vi "ep_Read Current Channels.vi"(8 "error in (no error)":errorcluster, 11 "system info in":refnum<class "EP System Info.lvclass">) -> (0 "error out":errorcluster, 2 "current channels":T1[](array[typedef]) {"physical channels"."channel phase" items=["Phase A (L1)", "Phase B (L2)", "Phase C (L3)", "Phase N (Neutral)"]}, 3 "system info out":refnum<class "EP System Info.lvclass">)   [LabVIEW 2014, in "NI_EP_Power Quality.lvlib" / "EP System Info.lvclass"]
uses:
  <vilib>/addons/Electrical Power/PQ/Common/Classes/System Info/EP System Info.lvclass
  <vilib>/addons/Electrical Power/PQ/Common/Controls/ep_Channels Config.ctl
  <vilib>/addons/Electrical Power/PQ/Common/Controls/ep_Channel Phase.ctl
  <vilib>/addons/Electrical Power/PQ/Common/Classes/System Info/EP System Info.lvclass/EP System Info.ctl
  <vilib>/addons/Electrical Power/PQ/NI_EP_Power Quality.lvlib
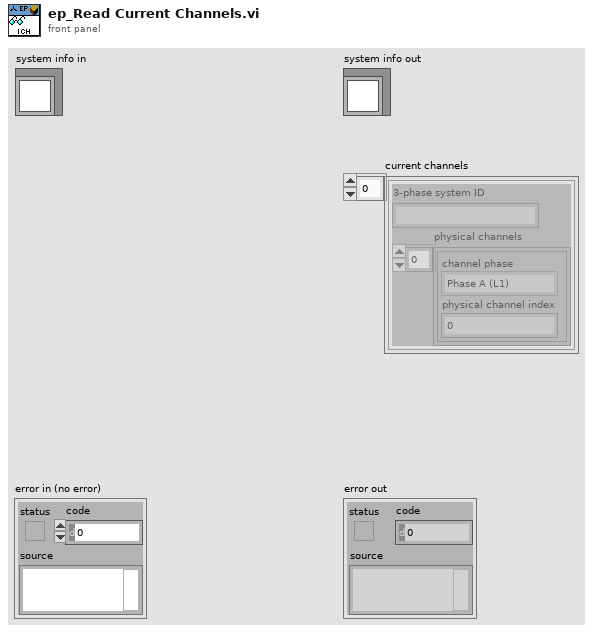
[diagram p1: front panel]
types:
  T1 = typedef "NI_EP_Power Quality.lvlib/ep_Channels Config.ctl" = cluster{"3-phase system ID":string, "physical channels":cluster{"channel phase":T2, "physical channel index":u16}[]}
  T2 = typedef "NI_EP_Power Quality.lvlib/ep_Channel Phase.ctl" = u16
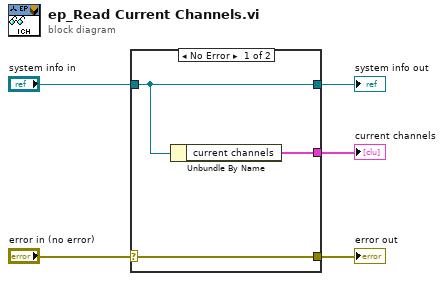
[diagram p0: block diagram]
diagram:
  n1 = case shown="No Error" "error in (no error)" {
    selector: "error in (no error)" -> [w8 w9]
    tunnel: [w8 w9] -> w4
    tunnel: [w7 w10] -> w2
    tunnel: "system info in" -> [w7 w10]
    tunnel: [w6 _] -> w1
    frame No Error {
      n2 = Unbundle By Name(w7) -> ("current channels"=w6:T1[])
    }
    frame Error {
    }
  }
  "error out" <- w4
  "system info out" <- w2
  "current channels" <- w1
